vi "List All Valid Notifiers.vi"(8 "error in (no error)":errorcluster, 11 "SMO":refnum<class "SMO.lvclass">) -> (0 "error out":errorcluster, 2 "Valid Notifiers":refnum<notifier>[](array[refnum]), 3 "SMO out":refnum<class "SMO.lvclass">)   [LabVIEW 2013, in "SMO.lvclass"]
uses:
  SMO.lvclass
  SMO.lvclass/SMO.ctl
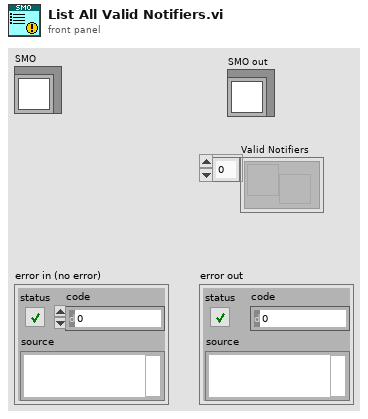
[diagram p1: front panel]
types:
  T1 = typedef "SMO.lvclass/PrivateData--Ref.ctl" = refnum<data-value>
  T2 = typedef "SMO.lvclass/PrivateData--Cluster.ctl" = cluster{"SMO Name":string, "Parent Call":T3, "Registered Processes":T4[], "Sync Notifier":refnum<notifier>, "Process Error Notifier":refnum<notifier>, "Protected Events":T5, "Public Events":T6, "SMO State":T7}
  T3 = typedef "SMO.lvclass/Parent Call--Enum.ctl" = enum16{"Allows parent to run", "Does not request parent to run"}
  T4 = typedef "SMO.lvclass/RegisteredProcessData--Cluster.ctl" = cluster{"Name":string, "Static VI Ref":refnum<vi>, "Running":bool, "NotifierRef":u32}
  T5 = typedef "SMO.lvclass/Protected Events.ctl" = cluster{"StopProcesses":refnum<user-event>, "AbortProcesses":refnum<user-event>}
  T6 = typedef "SMO.lvclass/Public Events.ctl" = cluster{"Error":refnum<user-event>, "State":refnum<user-event>}
  T7 = typedef "SMO.lvclass/SMOState --Enum.ctl" = enum16{"unknown", "Created", "Started", "Stopped"}
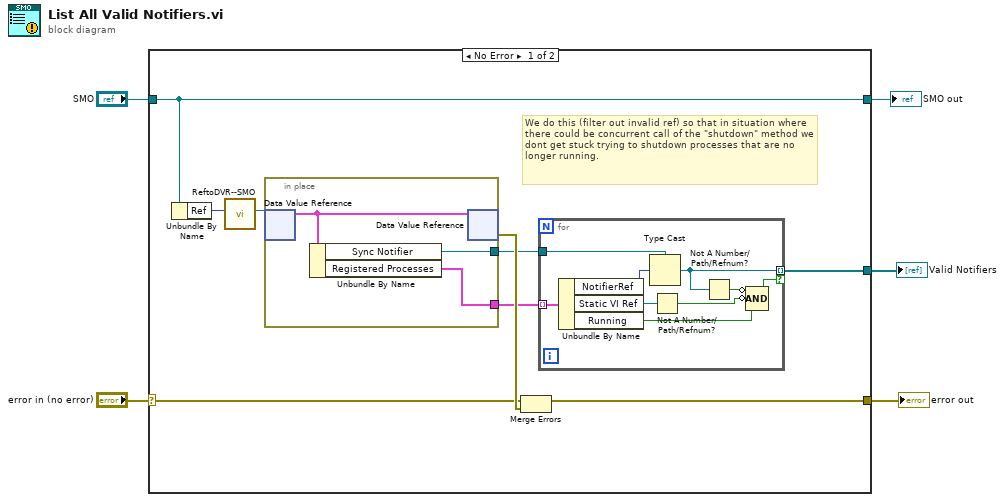
[diagram p0: block diagram]
diagram:
  n1 = case shown="No Error" "error in (no error)" {
    selector: "error in (no error)" -> [w6 w27]
    tunnel: [w14 w27] -> w5
    tunnel: [w12 _] -> w4
    tunnel: "SMO" -> [w7 w28]
    tunnel: [w7 w28] -> w2
    frame No Error {
      # "We do this (filter out invalid ref) so that in situation where there could be concurrent call of the \"shutdown\" method we dont get stuck trying to shutdown processes that are no longer running."
      n2 = Unbundle By Name(w7) -> ("Ref"=w9:u32)
      n3 = call "ReftoDVR--SMO.vi"("Ref"=w9) -> ("Ref"=w10:T1)  [unwired: 10 in]
      n4 = in-place {
        in-place-border: [w25] -> w8
        in-place-border: [w24] -> w11
        n5 = in-place-dvr #1(w10) -> (w26:T2)  [unwired: 1 out]
        n6 = Unbundle By Name(w26) -> ("Sync Notifier"=w24:refnum<notifier>, "Registered Processes"=w25:T4[])
        n7 = in-place-dvr #1(w26) -> (w13:errorcluster)  [unwired: 1 out]
      }
      n8 = Merge Errors(w6, w13) -> (w14:errorcluster)
      n9 = for {
        tunnel: w8 -> [w23] mode=indexing
        tunnel: [w19] -> w12 mode=indexing if=w15
        tunnel: w11 -> [w21]
        n10 = Unbundle By Name(w23) -> ("NotifierRef"=w20:u32, "Static VI Ref"=w22:refnum<vi>, "Running"=w16:bool)
        n11 = Type Cast(type=w21, x=w20) -> (*(type *) &x=w19:refnum<notifier>)
        n12 = Not A Number/Path/Refnum?(number/path/refnum=w22) -> (NaN/Path/Refnum?=w17:bool)
        n13 = Not A Number/Path/Refnum?(number/path/refnum=w19) -> (NaN/Path/Refnum?=w18:bool)
        n14 = Compound Arithmetic op=AND(invert w18, invert w17, w16) -> (w15:bool)
      }
    }
    frame Error {
    }
  }
  "error out" <- w5
  "Valid Notifiers" <- w4
  "SMO out" <- w2
